vi "4p1_HW_Task2B_jones6sv.vi"() -> ()   [LabVIEW 2016]
uses:
  <vilib>/express/express arith-compare/Formula/XNode/ExpressFormulaBlockNode.xnode
panel:
  out "Max Range":dbl
  out "Max height":dbl
  out "Time of Impact":dbl
  in  "Velocity":dbl
  in  "Angle":dbl
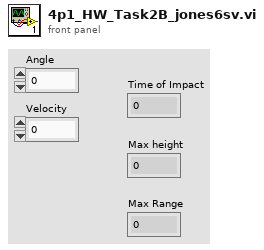
[diagram p1: front panel]
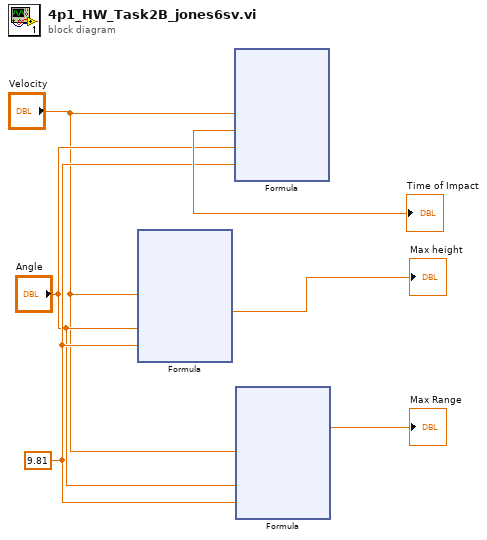
[diagram p0: block diagram]
diagram:
  w5 = 9.81
  n1 = xnode "Formula"("Velocity"="Velocity", "Angle"="Angle", "Gravity"=w5) -> ("Result"=→"Max height":dbl)  [unwired: 1 in, 1 out]
  n2 = xnode "Formula"("Velocity"="Velocity", "Angle"="Angle", "Gravity"=w5) -> ("Result"=→"Time of Impact":dbl)  [unwired: 1 in, 1 out]
  n3 = xnode "Formula"("Velocity"="Velocity", "Angle"="Angle", "Gravity"=w5) -> ("Result"=→"Max Range":dbl)  [unwired: 1 in, 1 out]
